vi "PAS Control.vi"(11 "Events":refnum<event-registration>) -> ()   [LabVIEW 2012]
uses:
  Data/cPAS Cell Data/cPAS Cell Data.lvclass
  Reusable/PAS/Data/Cell/PAS Cell Data.lvclass
  Data/cPAS Data.lvclass
  Interface/Controls/PAS_MFC_SP.ctl
  Interface/Controls/pasCellTEC.ctl
  Interface/Controls/pasTECen.ctl
  Reusable/PAS/Main/Controls/Laser Modulation.ctl
  Utilities/FPGA/Controls/FPGAConfig.ctl
  Interface/Controls/pasLasCtl.ctl
panel:
  in  "pasLasCtl":T1 caption="Laser Control" {"Laser Output"."Span"."ch 5" min=0 max=20; "Laser Output"."Span"."ch 4" min=0 max=20; "Laser Output"."Span"."ch 3" min=0 max=20; "Laser Output"."Span"."ch 2" min=0 max=20; "Laser Output"."Span"."ch 1" min=0 max=20; "f0"."Cell 1" min=0 max=2000 step=1; "f0"."Cell 2" min=0 max=2000 step=1; "f0"."Cell 3" min=0 max=2000 step=1; "f0"."Cell 4" min=0 max=2000 step=1; "f0"."Cell 5" min=0 max=2000 step=1}
  out "PASCellT2":T4 caption="Thermistor Cell Temperature (degC)" {"Cell 5" format="%.2f"; "Cell 4" format="%.2f"; "Cell 3" format="%.2f"; "Cell 2" format="%.2f"; "Cell 1" format="%.2f"}
  out "tecP":sgl caption="TEC Power (%)" format="%#.2f"
  in  "pas::rhctl":bool caption="RH Control"
  in  "pas::rh":dbl caption="RH (%)"
  in  "ptecHumEn":bool caption="Enable"
  in  "pas::satT":sgl caption="T(degC)"
  out "PASCellT":T5 caption="TEC Thermistor Cell Temperature (degC)" {"Cell 5" format="%.2f"; "Cell 4" format="%.2f"; "Cell 3" format="%.2f"; "Cell 2" format="%.2f"; "Cell 1" format="%.2f"}
  out "pasRH":T6 caption="Vaisala Data" {"c 5"."TRH" format="%#.2f"; "c 5"."RH" format="%#.2f"; "c 4"."TRH" format="%#.2f"; "c 4"."RH" format="%#.2f"; "c 3"."TRH" format="%#.2f"; "c 3"."RH" format="%#.2f"; "c 2"."TRH" format="%#.2f"; "c 2"."RH" format="%#.2f"; "c 1"."TRH" format="%#.2f"; "c 1"."RH" format="%#.2f"}
  out "pasACat":T7 caption="Alicat Data" {"c 5 2"."P" format="%.2f"; "c 5 2"."T" format="%.2f"; "c 5 2"."Q" format="%.2f"; "c 4"."P" format="%.2f"; "c 4"."T" format="%.2f"; "c 4"."Q" format="%.2f"; "c 3"."P" format="%.2f"; "c 3"."T" format="%.2f"; "c 3"."Q" format="%.2f"; "c 2"."P" format="%.2f"; "c 2"."T" format="%.2f"; "c 2"."Q" format="%.2f"; "c 1"."P" format="%.2f"; "c 1"."T" format="%.2f"; "c 1"."Q" format="%.2f"}
  out "pasTte":sgl caption="TEC Temperature\n(degC)" format="%#.2f"
  in  "pasTECEn":T8 caption="Enable TECs"
  in  "pasTcell":T9 caption="Temperature \n (degC)"
  in  "pasFlows":T10 caption="Flow Rate Setpoint (LPM)" {"Cell 5" min=0 max=5; "Cell 4" min=0 max=5; "Cell 3" min=0 max=5; "Cell 2" min=0 max=5; "Cell 1" min=0 max=5}
  in  "pasTteSP":sgl caption="TEC Temperature \nSetpoint (degC)" format="%#.2f"
  out "Thum":sgl caption="Tsat\n(degC)" format="%#.2g"
  # "PAS Housekeeping Data"
  # "PAS Controls"
  # "TEC Temperature Control"
  # "RH Control"
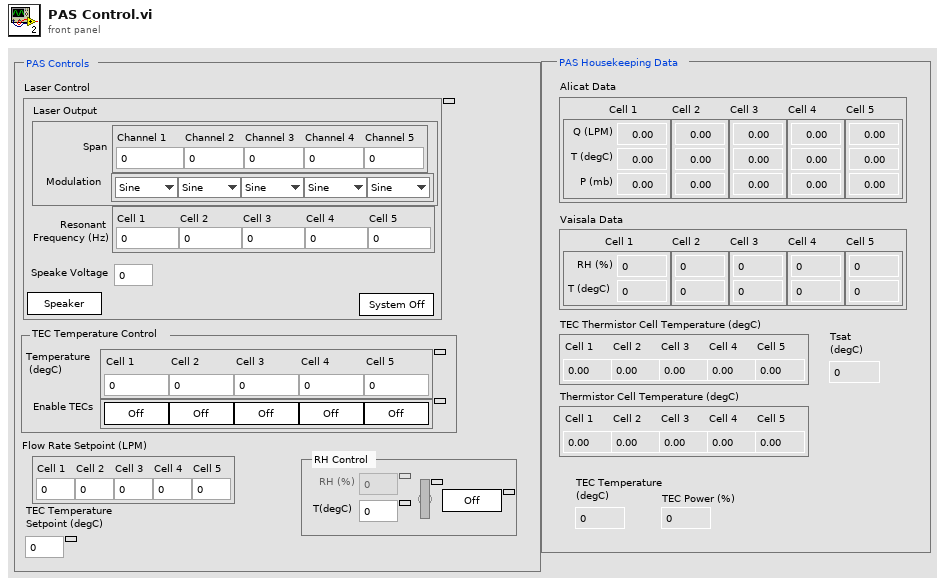
[diagram p1: front panel]
types:
  T1 = typedef "pasLasCtl.ctl" = cluster{"Laser Output":T2, "f0":cluster{"Cell 1":sgl, "Cell 2":sgl, "Cell 3":sgl, "Cell 4":sgl, "Cell 5":sgl}, "drive":bool, "lasSysPow":bool, "Speake Voltage":dbl}
  T2 = typedef "FPGAConfig.ctl" = cluster{"Span":cluster{"ch 1":sgl, "ch 2":sgl, "ch 3":sgl, "ch 4":sgl, "ch 5":sgl}, "mod":cluster{"ch 1":T3, "ch 2":T3, "ch 3":T3, "ch 4":T3, "ch 5":T3}}
  T3 = typedef "Laser Modulation.ctl" = enum8{"Sine", "Square"}
  T4 = cluster{"[0]":sgl, "[1]":sgl, "[2]":sgl, "[3]":sgl, "[4]":sgl}
  T5 = cluster{"ScaledData[0]":sgl, "ScaledData[1]":sgl, "ScaledData[2]":sgl, "ScaledData[3]":sgl, "ScaledData[4]":sgl}
  T6 = cluster{"c 1":cluster{"RH":sgl, "TRH":sgl}, "c 2":cluster{"RH":sgl, "TRH":sgl}, "c 3":cluster{"RH":sgl, "TRH":sgl}, "c 4":cluster{"RH":sgl, "TRH":sgl}, "c 5":cluster{"RH":sgl, "TRH":sgl}}
  T7 = cluster{"c 1":cluster{"Q":sgl, "T":sgl, "P":sgl}, "c 2":cluster{"Q":sgl, "T":sgl, "P":sgl}, "c 3":cluster{"Q":sgl, "T":sgl, "P":sgl}, "c 4":cluster{"Q":sgl, "T":sgl, "P":sgl}, "c 5 2":cluster{"Q":sgl, "T":sgl, "P":sgl}}
  T8 = typedef "pasTECen.ctl" = cluster{"Cell 1":bool, "Cell 2":bool, "Cell 3":bool, "Cell 4":bool, "Cell 5":bool}
  T9 = typedef "pasCellTEC.ctl" = cluster{"Cell 1":sgl, "Cell 2":sgl, "Cell 3":sgl, "Cell 4":sgl, "Cell 5":sgl}
  T10 = typedef "PAS_MFC_SP.ctl" = cluster{"Cell 1":sgl, "Cell 2":sgl, "Cell 3":sgl, "Cell 4":sgl, "Cell 5":sgl}
  T11 = enum8{"Enabled", "Disabled", "Disabled and Grayed Out"}
  T12 = cluster{"[0]":cluster{"Q":sgl, "T":sgl, "P":sgl}, "[1]":cluster{"Q":sgl, "T":sgl, "P":sgl}, "[2]":cluster{"Q":sgl, "T":sgl, "P":sgl}, "[3]":cluster{"Q":sgl, "T":sgl, "P":sgl}, "[4]":cluster{"Q":sgl, "T":sgl, "P":sgl}}
  T13 = cluster{"Input 1":sgl, "Input 2":sgl, "Power":sgl}
  T14 = cluster{"T":sgl, "TRH":sgl, "RH":sgl, "laserRMS":sgl}
  T15 = cluster{"[0]":cluster{"RH":sgl, "TRH":sgl}, "[1]":cluster{"RH":sgl, "TRH":sgl}, "[2]":cluster{"RH":sgl, "TRH":sgl}, "[3]":cluster{"RH":sgl, "TRH":sgl}, "[4]":cluster{"RH":sgl, "TRH":sgl}}
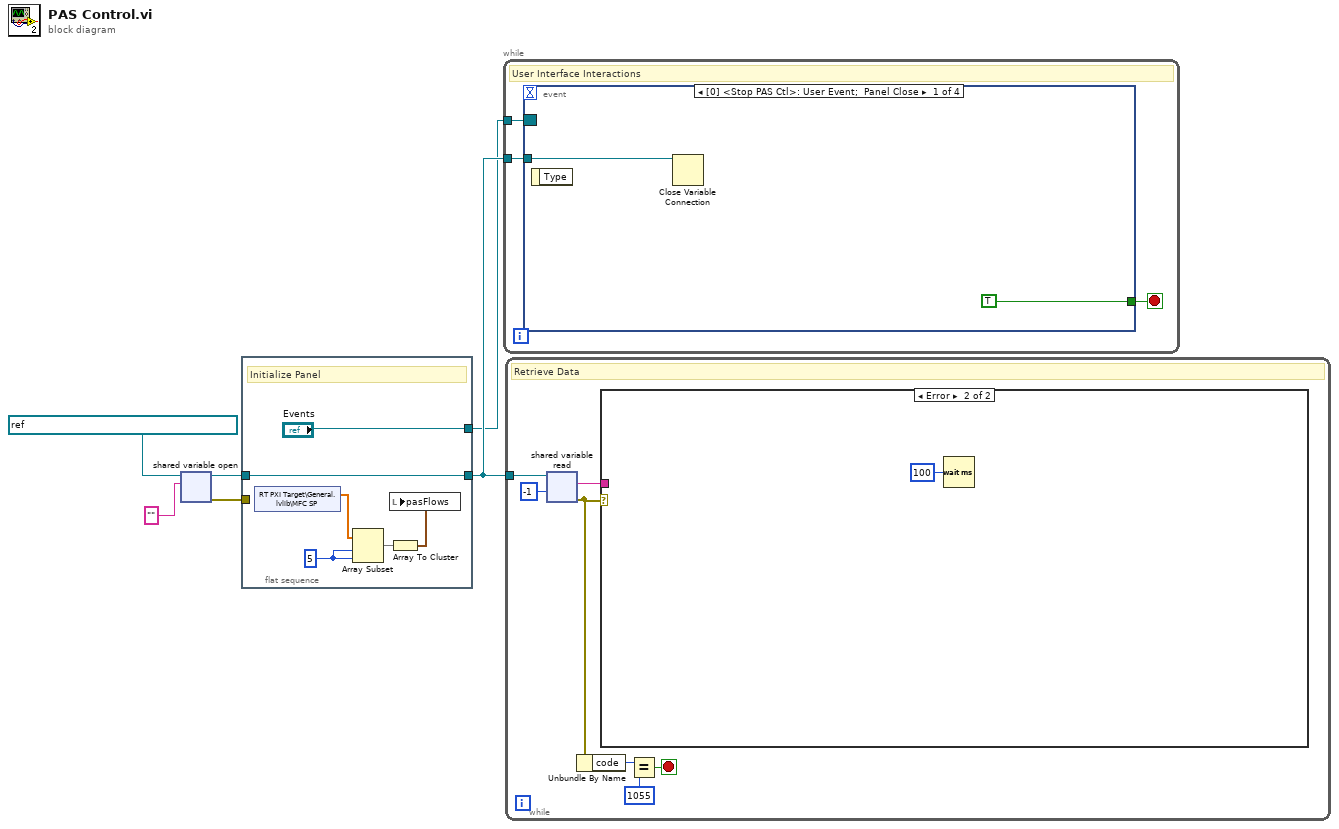
[diagram p0: block diagram]
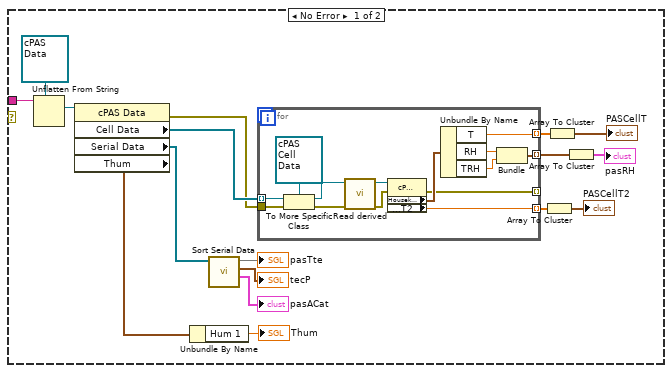
[diagram p2: hidden frame]
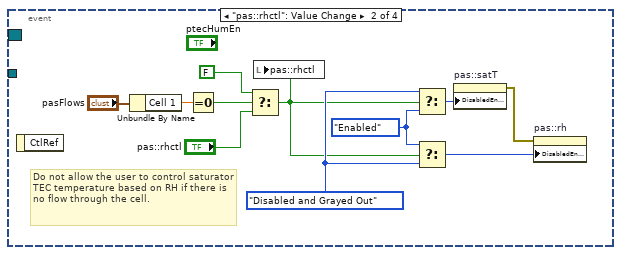
[diagram p3: hidden frame]
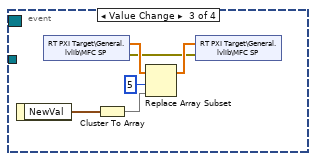
[diagram p4: hidden frame]
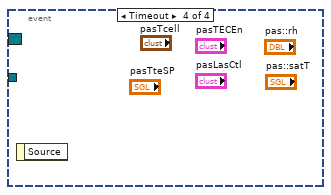
[diagram p5: hidden frame]
diagram:
  n1 = shared-variable-open(refnum<k21> "ni.var.psp://rt pxi target/PAS_Var/Data" ("shared variable refnum in"), "") -> (w4:refnum<k21>, w2:errorcluster)  [unwired: 2 in]
  n2 = flat-sequence {
    tunnel: w4 -> [w8]
    tunnel: [w8] -> w3
    tunnel: w2 -> [_]
    tunnel: ["Events"] -> w1
    frame #0 {
      w11 = 5 ("length")
      # "Initialize Panel"
      n3 = shared-variable "RT PXI Target\\General.lvlib\\MFC SP"() -> (w12:sgl[])  [unwired: 1 in, 1 out]
      n4 = Array Subset(array=w12, index=w11, length=w11) -> (w10:sgl[])
      n5 = Array To Cluster(array=w10) -> (cluster=w9:T4)
      n6 = local write "pasFlows"(w9) -> ()
    }
  }
  n7 = while {
    tunnel: w3 -> [w14]
    tunnel: w1 -> [w15]
    stop <- w13 stop-if-true
    # "User Interface Interactions"
    n8 = event shown="[0] <Stop PAS Ctl>: User Event;  Panel Close" {
      selector: w15 -> [_ _ _ _]
      dyn-events: _ -> [_ _ _ _]
      timeout: _ -> [_ _ _ _]
      tunnel: w14 -> [w17 _ _ _]
      tunnel: [TRUE _ _ _] -> w13
      event User Event; Panel Close {
        n9 = event-data() -> ()  [unwired: 1 in, 1 out]
        n10 = Close Variable Connection(11:w17) -> ()  [unwired: 1 in, 1 out]
      }
      event "pas::rhctl": Value Change {
        w26 = T11."Disabled and Grayed Out" ("Disabled")
        w27 = T11."Enabled" ("Disabled")
        # "Do not allow the user to control saturator TEC temperature based on RH if there is no flow through the cell."
        n11 = event-data() -> ()  [unwired: 1 in, 1 out]
        n12 = Unbundle By Name("pasFlows") -> ("Cell 1"=w19:sgl)
        n13 = Equal To 0?(x=w19) -> (x = 0?=w23:bool)
        n14 = Select(t=FALSE, s=w23, f="pas::rhctl") -> (s? t:f=w21:bool)
        n15 = local write "pas::rhctl"(w21) -> ()
        n16 = Select(t=w26, s=w21, f=w27) -> (s? t:f=w25:T11)
        n17 = Select(t=w27, s=w21, f=w26) -> (s? t:f=w28:T11)
        n18 = property on="pas::satT" class="DigNum (strict)"("DisabledEnum"=w25) -> (error out=w24:errorcluster)  [unwired: 2 in, 1 out]
        n19 = property on="pas::rh" class="DigNum (strict)"(error in=w24, "DisabledEnum"=w28) -> ()  [unwired: 1 in, 2 out]
      }
      event Value Change {
        n20 = event-data() -> ("NewVal"=w33:T10)  [unwired: 1 in]
        n21 = shared-variable "RT PXI Target\\General.lvlib\\MFC SP"() -> (w34:sgl[], error out=w29:errorcluster)  [unwired: 1 in]
        n22 = Cluster To Array(cluster=w33) -> (array=w32:sgl[])
        n23 = Replace Array Subset(array=w34, new element=w32, index=5) -> (w30:sgl[])
        n24 = shared-variable "RT PXI Target\\General.lvlib\\MFC SP"(w30, error in=w29) -> ()  [unwired: 1 out]
      }
      event Timeout {
        n25 = event-data() -> ()  [unwired: 1 in, 1 out]
      }
    }
  }
  n26 = while {
    tunnel: w3 -> [w41]
    stop <- w37 stop-if-true
    # "Retrieve Data"
    n27 = shared-variable-read(w41, -1 ("timeout ms")) -> (w38:errorcluster, w39:string)  [unwired: 1 in, 3 out]
    n28 = Unbundle By Name(w38) -> ("code"=w36:i32)
    n29 = case shown="Error" w38 {
      tunnel: w39 -> [w54 _]
      frame No Error {
        n30 = Unflatten From String(type=refnum<class "cPAS Data.lvclass"> refnum ("cPAS Data"), binary string=w54) -> (value=w50:refnum<class "cPAS Data.lvclass">)  [unwired: 3 in, 2 out]
        n31 = property class="cPAS Data"(reference=w50) -> (error out=w48:errorcluster, "Cell Data"=w49:refnum<class "PAS Cell Data.lvclass">[], "Serial Data"=w47:refnum<class "Data.lvclass">[], "Thum"=w43:cluster{"Hum 1":sgl, "Hum 2":sgl})  [unwired: 1 in, 1 out]
        n32 = Unbundle By Name(w43) -> ("Hum 1"=→"Thum":sgl)
        n33 = call "Sort Serial Data.vi"("SerialData"=w47) -> ("acatDataOut"=→"pasACat":T12, "TEC Data"=→"tecP":T13, 3:→"pasTte")  [unwired: 7 in, 1 out]
        n34 = for {
          tunnel: w49 -> [w62] mode=indexing
          tunnel: [w69] -> w55 mode=indexing
          tunnel: [w70] -> w56 mode=indexing
          tunnel: w48 -> [w65]
          tunnel: [w60] -> _ mode=indexing
          tunnel: [w59] -> w52 mode=indexing
          n35 = To More Specific Class(target class=refnum<class "cPAS Cell Data.lvclass"> refnum ("cPAS Cell"), reference=w62, error in=w65) -> (specific class reference=w61:refnum<class "cPAS Cell Data.lvclass">, error out=w64:errorcluster)
          n36 = call "Read derived.vi"("error in"=w64, "PAS Cell Data in"=w61) -> ("error out"=w72:errorcluster, "PAS Cell Data out"=w67:refnum<class "cPAS Cell Data.lvclass">)  [unwired: 7 in, 1 out]
          n37 = property class="cPAS Cell"(reference=w67, error in=w72) -> (error out=w60:errorcluster, "Housekeeping"=w66:T14, "Data Access:T2"=w59:sgl)  [unwired: 1 out]
          n38 = Unbundle By Name(w66) -> ("T"=w69:sgl, "RH"=w68:sgl, "TRH"=w71:sgl)
          n39 = Bundle("RH"=w68, "TRH"=w71) -> (w70:cluster{"RH":sgl, "TRH":sgl})  [unwired: 1 in]
        }
        n40 = Array To Cluster(array=w52) -> (cluster=→"PASCellT2":T4)
        n41 = Array To Cluster(array=w55) -> (cluster=→"PASCellT":T4)
        n42 = Array To Cluster(array=w56) -> (cluster=→"pasRH":T15)
      }
      frame Error {
        n43 = Wait (ms)(milliseconds to wait=u32 100) -> ()  [unwired: 1 out]
      }
    }
    n44 = Equal?(x=w36, y=1055 ("x")) -> (x = y?=w37:bool)
  }
